vi "main backup.vi"() -> ()   [LabVIEW 2013]
panel:
  out "输出数组":i32[][](array[numeric])
  out "强度图":i32[][](graph)
  in  "数组":i32[](array[numeric])
  in  "Camera Control":bool
  in  "Trigger":bool
  out "Frame Rate":sgl
  in  "?":bool
  in  "Stop Grabbing":bool
  out "# of Iteration":i32
  in  "Live Image Display":refnum<k7>(container)
  # "This is an simlple ActiveX example using methods provided by ActiveFlyCapConctrol to grab images from an PGR camera,  \ndisplay it on the screen and retrieve the frame rate at the same time. Also, it can toggle between free running mode and software\ntrigger mode. It is meant to let new users become farmiliar with the ActiveX control provided by the Flycapture SDK, so more compilcated blocks can be build upon."
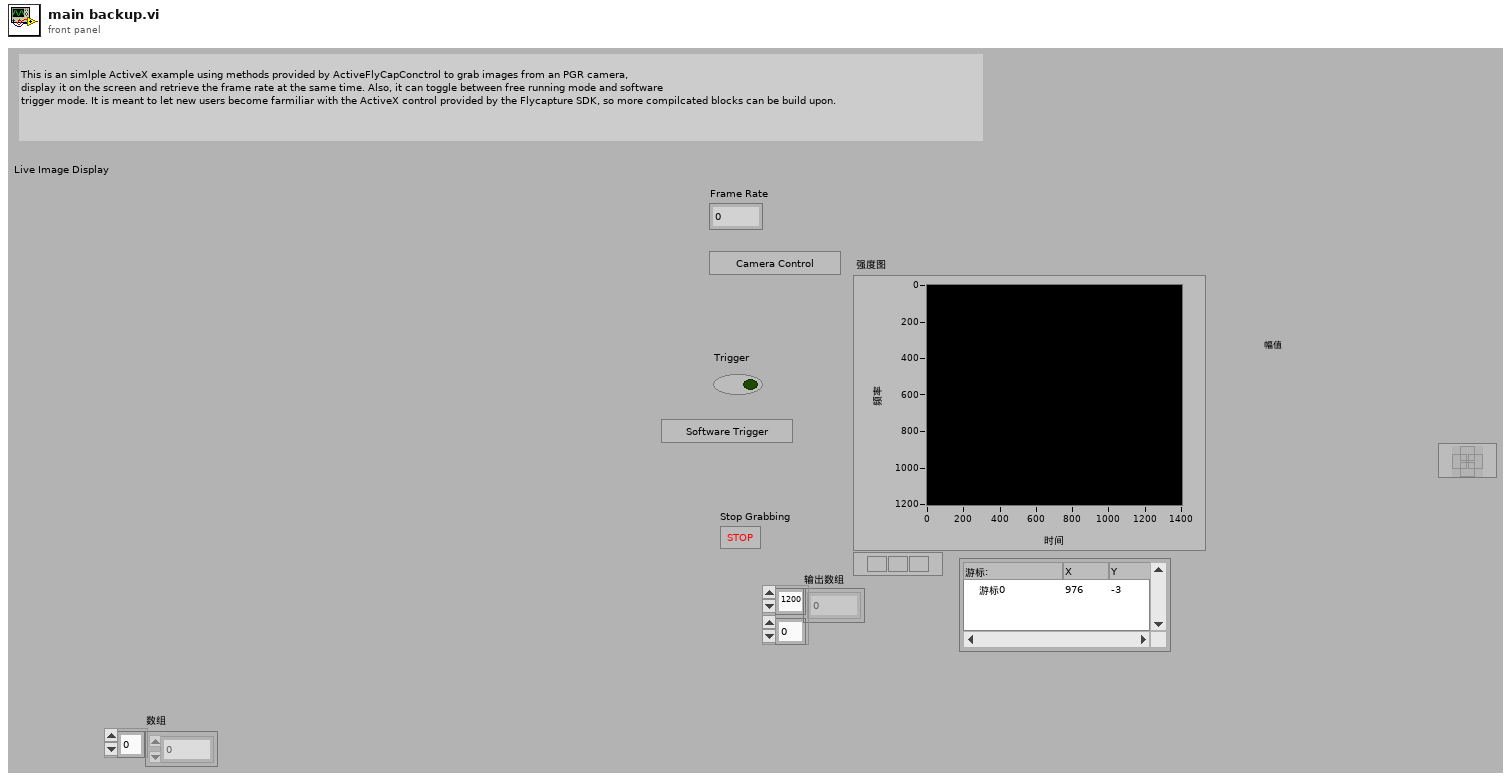
[diagram p1: front panel]
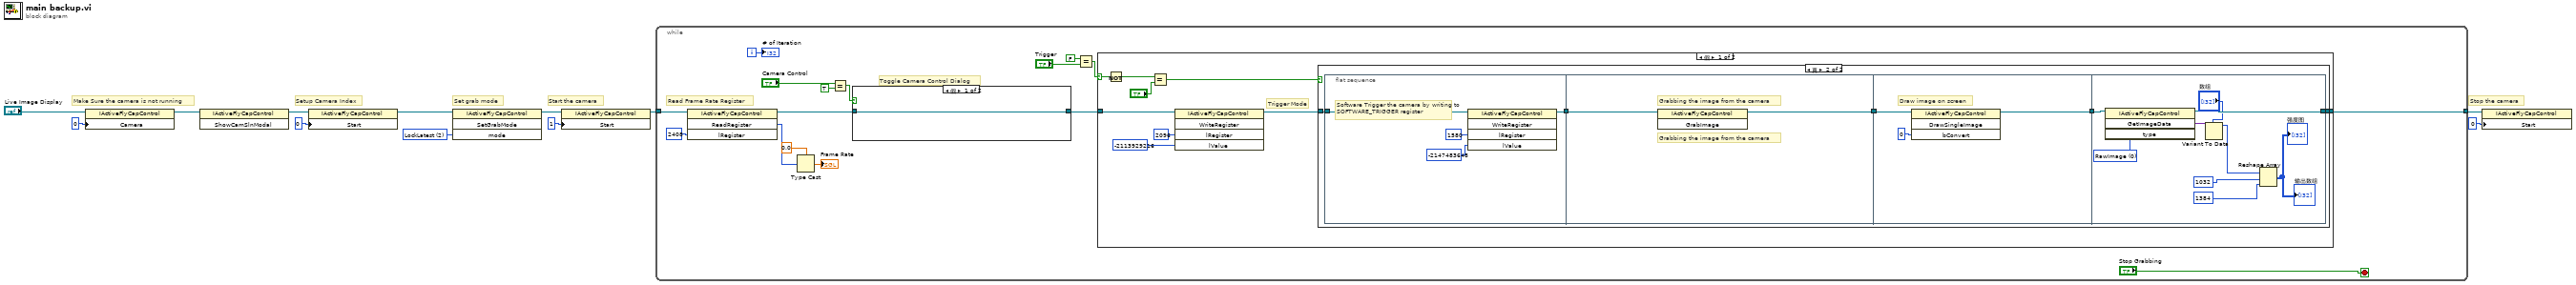
[diagram p0: block diagram]
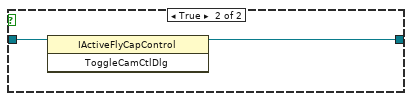
[diagram p2: hidden frame]
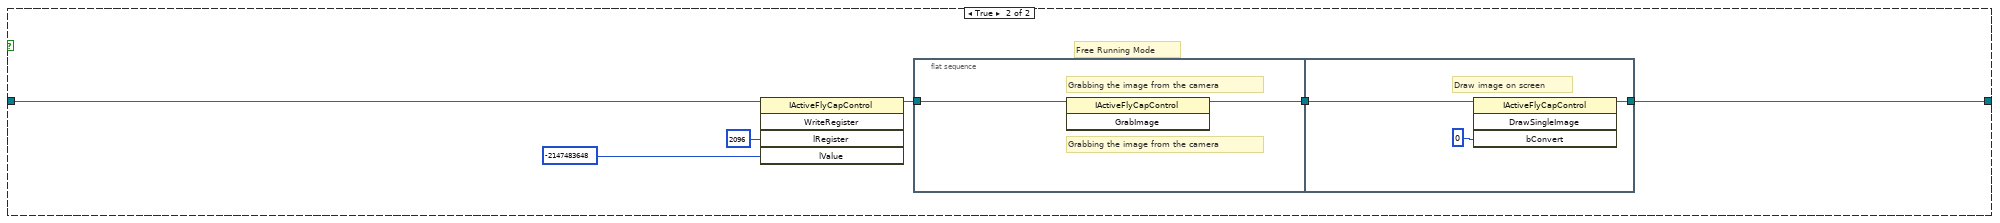
[diagram p4: hidden frame]
diagram:
  w1 = 2 items=["FreeRunning", "LockNext", "LockLatest"] ("mode")
  # "Start the camera"
  # "Stop the camera"
  # "Setup Camera Index"
  # "Set grab mode"
  # "Make Sure the camera is not running"
  n1 = property class="IActiveFlyCapControl"(reference="Live Image Display", "Camera"=0 ("Start")) -> (reference out=w8:refnum<k7>)  [unwired: 1 in, 1 out]
  n2 = invoke class="IActiveFlyCapControl" method="ShowCamSlnModal"(reference=w8) -> (reference out=w7:refnum<k7>)  [unwired: 2 in, 2 out]
  n3 = property class="IActiveFlyCapControl"(reference=w7, "Start"=0 ("Camera")) -> (reference out=w9:refnum<k7>)  [unwired: 1 in, 1 out]
  n4 = invoke class="IActiveFlyCapControl" method="SetGrabMode"(reference=w9, "mode"=w1) -> (reference out=w2:refnum<k7>)  [unwired: 2 in, 3 out]
  n5 = property class="IActiveFlyCapControl"(reference=w2, "Start"=1) -> (reference out=w3:refnum<k7>)  [unwired: 1 in, 1 out]
  n6 = while {
    tunnel: w3 -> [w24]
    tunnel: [w13] -> w4
    i -> [w27]
    stop <- "Stop Grabbing" stop-if-true
    # "Read Frame Rate Register"
    # "Toggle Camera Control Dialog"
    n7 = invoke class="IActiveFlyCapControl" method="ReadRegister"(reference=w24, "lRegister"=2408) -> (reference out=w18:refnum<k7>, "ReadRegister"=w21:u32)  [unwired: 2 in, 2 out]
    n8 = Type Cast(type=sgl 0.0 ("32-bit IEEE 754"), x=w21) -> (*(type *) &x=→"Frame Rate":sgl)
    n9 = Equal?(x="Camera Control", y=TRUE) -> (x = y?=w15:bool)
    n10 = case shown="假" w15 {
      tunnel: w18 -> [w29 w31]
      tunnel: [w29 w30] -> w14
      frame False {
      }
      frame True {
        n11 = invoke class="IActiveFlyCapControl" method="ToggleCamCtlDlg"(reference=w31) -> (reference out=w30:refnum<k7>)  [unwired: 2 in, 2 out]
      }
    }
    n12 = Equal?(x=FALSE, y="Trigger") -> (x = y?=w25:bool)
    n13 = case shown="假" w25 {
      selector: w25 -> [w39 _]
      tunnel: [w40 w69] -> w13
      tunnel: w14 -> [w33 w66]
      frame False {
        # "Trigger Mode"
        n14 = Not(x=w39) -> (.not. x?=w38:bool)
        n15 = Equal?(x=w38, y="?") -> (x = y?=w36:bool)
        n16 = invoke class="IActiveFlyCapControl" method="WriteRegister"(reference=w33, "lRegister"=2096, "lValue"=-2113929216 ("Register value in Hex 2")) -> (reference out=w32:refnum<k7>)  [unwired: 2 in, 4 out]
        n17 = case shown="真" w36 {
          tunnel: [w41 w44] -> w40
          tunnel: w32 -> [w41 w43]
          frame False {
          }
          frame True {
            n18 = flat-sequence {
              tunnel: [w48] -> w46
              tunnel: w43 -> [w47]
              tunnel: [w51] -> w45
              tunnel: w46 -> [w52]
              tunnel: w45 -> [w55]
              tunnel: [w53] -> w42
              tunnel: [w63] -> w44
              tunnel: w42 -> [w64]
              frame #0 {
                # "Software Trigger the camera by writing to SOFTWARE_TRIGGER register"
                n19 = invoke class="IActiveFlyCapControl" method="WriteRegister"(reference=w47, "lRegister"=1580, "lValue"=-2147483648 ("Register value in Hex 2")) -> (reference out=w48:refnum<k7>)  [unwired: 2 in, 4 out]
              }
              frame #1 {
                # "Grabbing the image from the camera"
                # "Grabbing the image from the camera"
                n20 = invoke class="IActiveFlyCapControl" method="GrabImage"(reference=w52) -> (reference out=w51:refnum<k7>)  [unwired: 2 in, 2 out]
              }
              frame #2 {
                # "Draw image on screen"
                n21 = invoke class="IActiveFlyCapControl" method="DrawSingleImage"(reference=w55, "bConvert"=0) -> (reference out=w53:refnum<k7>)  [unwired: 2 in, 3 out]
              }
              frame #3 {
                w62 = 0 items=["RawImage", "ColorProcessedImage"] ("type")
                n22 = invoke class="IActiveFlyCapControl" method="GetImageData"(reference=w64, "type"=w62) -> (reference out=w63:refnum<k7>, "GetImageData"=w61:variant)  [unwired: 2 in, 2 out]
                n23 = Variant To Data(type="数组", Variant=w61) -> (data=w59:i32[])  [unwired: 1 in, 1 out]
                n24 = Reshape Array(w59, 1032 ("维数大小"), 1384 ("维数大小")) -> (→"强度图" →"输出数组":i32[][])
              }
            }
          }
        }
      }
      frame True {
        # "Free Running Mode"
        n25 = invoke class="IActiveFlyCapControl" method="WriteRegister"(reference=w66, "lRegister"=2096, "lValue"=-2147483648 ("Register value in Hex 2")) -> (reference out=w65:refnum<k7>)  [unwired: 2 in, 4 out]
        n26 = flat-sequence {
          tunnel: [w72] -> w70
          tunnel: w65 -> [w71]
          tunnel: w70 -> [w75]
          tunnel: [w74] -> w69
          frame #0 {
            # "Grabbing the image from the camera"
            # "Grabbing the image from the camera"
            n27 = invoke class="IActiveFlyCapControl" method="GrabImage"(reference=w71) -> (reference out=w72:refnum<k7>)  [unwired: 2 in, 2 out]
          }
          frame #1 {
            # "Draw image on screen"
            n28 = invoke class="IActiveFlyCapControl" method="DrawSingleImage"(reference=w75, "bConvert"=0) -> (reference out=w74:refnum<k7>)  [unwired: 2 in, 3 out]
          }
        }
      }
    }
    "# of Iteration" <- w27
  }
  n29 = property class="IActiveFlyCapControl"(reference=w4, "Start"=0) -> ()  [unwired: 1 in, 2 out]
